vi "TETRIX Servos Move All_HT_myRIO.vi"(0 "Servo 4 (0 - 255)":u8(slide)=128 step=1 scale=0.0..255.0, 1 "Servo 5 (0 - 255)":u8(slide)=128 step=1 scale=0.0..255.0, 2 "Servo 6 (0 - 255)":u8(slide)=128 step=1 scale=0.0..255.0, 4 "Enable Sync: Fast | Medium | Slow | None":string(combo)="None", 5 "Controller Daisy Chain Position (1 - 4)":u8=1, 6 "Servo 3 (0 - 255)":u8(slide)=128 step=1 scale=0.0..255.0, 7 "Servo 2 (0 - 255)":u8(slide)=128 step=1 scale=0.0..255.0, 8 "Servo 1 (0 - 255)":u8(slide)=128 step=1 scale=0.0..255.0, 9 "error in (no error)":errorcluster) -> (3 "error out":errorcluster)   [LabVIEW 2014]
uses:
  <vilib>/myRIO/Instrument Drivers/Onboard IO/I2C/vis/Configure.vi
  <vilib>/myRIO/Instrument Drivers/Onboard IO/I2C/vis/Write.vi
  Global Servo Controls.vi
  <vilib>/myRIO/Instrument Drivers/Onboard IO/I2C/vis/Smart Open.vi
  <vilib>/Utility/error.llb/Error Cluster From Error Code.vi
  <vilib>/myRIO/Common/Instrument Driver Framework/myRIO v1.0/I2C/vis/myRIO v1.0 Configure I2C.vi
  <vilib>/myRIO/Common/Instrument Driver Framework/myRIO v1.0/I2C/vis/myRIO v1.0 Write I2C.vi
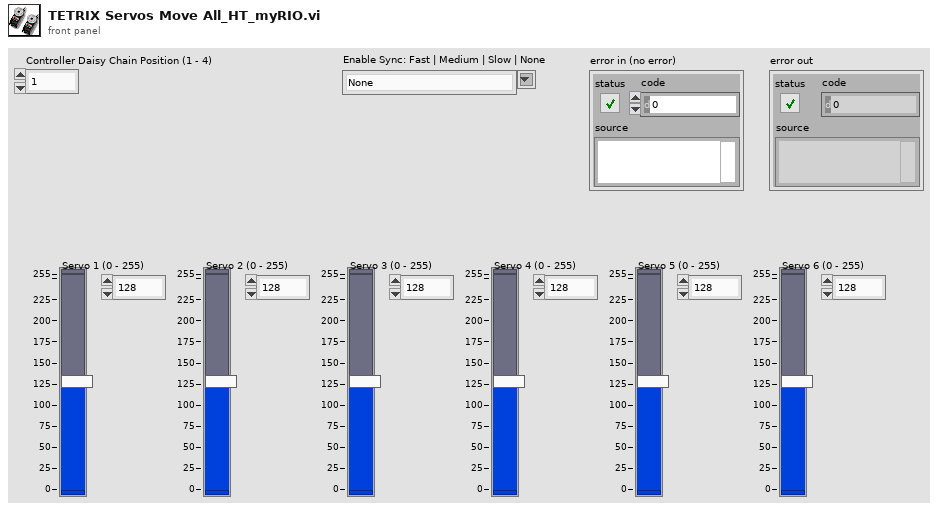
[diagram p1: front panel]
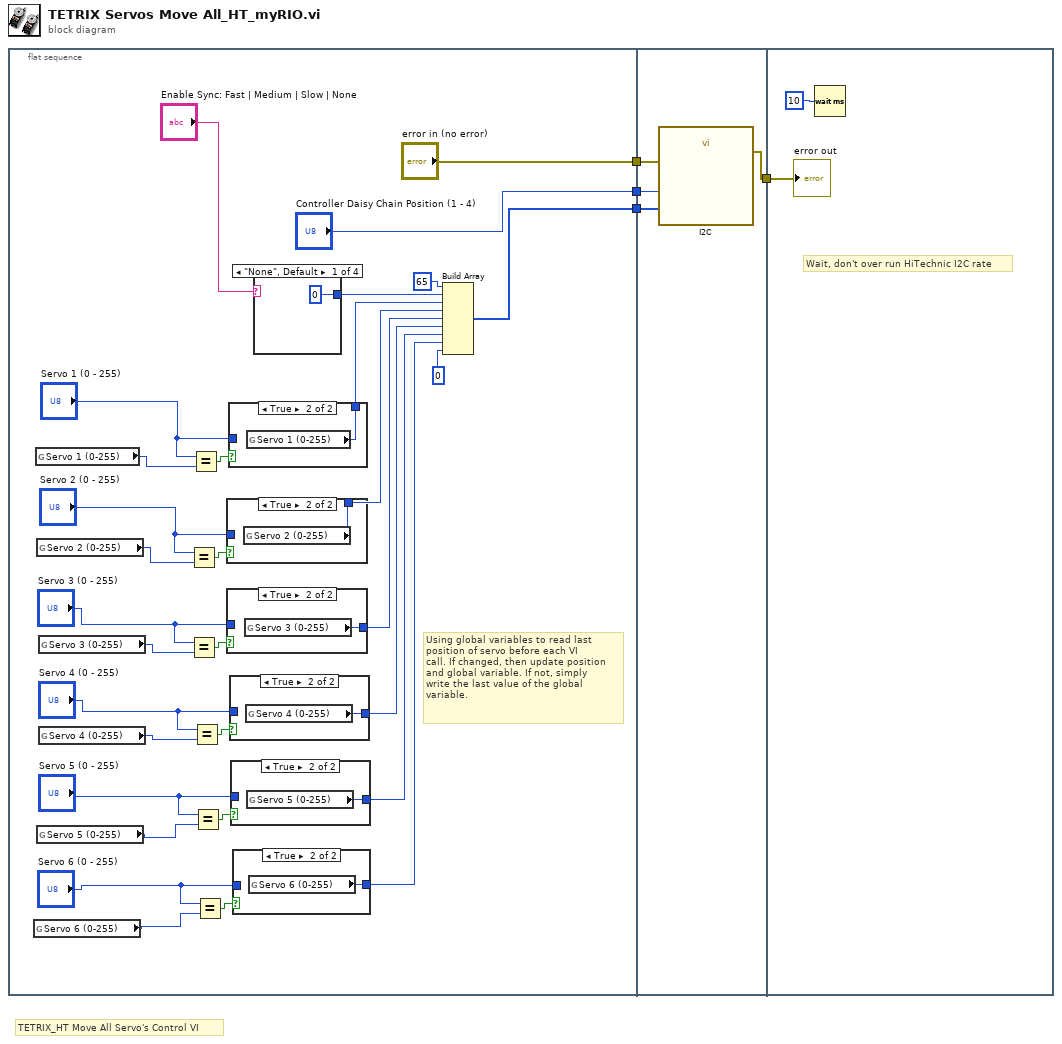
[diagram p0: block diagram]
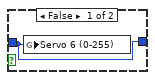
[diagram p2: hidden frame]
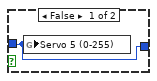
[diagram p3: hidden frame]
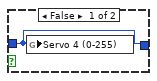
[diagram p4: hidden frame]
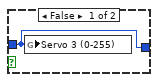
[diagram p5: hidden frame]
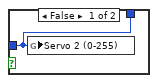
[diagram p6: hidden frame]
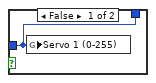
[diagram p7: hidden frame]
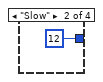
[diagram p8: hidden frame]
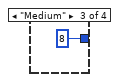
[diagram p9: hidden frame]
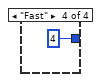
[diagram p10: hidden frame]
diagram:
  # "TETRIX_HT Move All Servo's Control VI"
  n1 = flat-sequence {
    tunnel: ["error in (no error)"] -> w4
    tunnel: ["Controller Daisy Chain Position (1 - 4)"] -> w3
    tunnel: [w29] -> w2
    tunnel: w4 -> [w55]
    tunnel: w3 -> [w54]
    tunnel: w2 -> [w53]
    tunnel: [w52] -> w1
    tunnel: w1 -> [w56]
    frame #0 {
      # "Using global variables to read last\nposition of servo before each VI\ncall. If changed, then update position\nand global variable. If not, simply\nwrite the last value of the global\nvariable."
      n2 = global read "Global Servo Controls.vi" "Servo 6 (0-255)"() -> (w14:u8)
      n3 = global read "Global Servo Controls.vi" "Servo 1 (0-255)"() -> (w10:u8)
      n4 = global read "Global Servo Controls.vi" "Servo 2 (0-255)"() -> (w18:u8)
      n5 = global read "Global Servo Controls.vi" "Servo 5 (0-255)"() -> (w15:u8)
      n6 = global read "Global Servo Controls.vi" "Servo 3 (0-255)"() -> (w17:u8)
      n7 = global read "Global Servo Controls.vi" "Servo 4 (0-255)"() -> (w16:u8)
      n8 = Equal?(x="Servo 2 (0 - 255)", y=w18) -> (x = y?=w27:bool)
      n9 = Equal?(x="Servo 3 (0 - 255)", y=w17) -> (x = y?=w26:bool)
      n10 = Equal?(x="Servo 1 (0 - 255)", y=w10) -> (x = y?=w28:bool)
      n11 = Equal?(x="Servo 4 (0 - 255)", y=w16) -> (x = y?=w24:bool)
      n12 = Equal?(x="Servo 5 (0 - 255)", y=w15) -> (x = y?=w22:bool)
      n13 = Equal?(x="Servo 6 (0 - 255)", y=w14) -> (x = y?=w20:bool)
      n14 = case shown="True" w27 {
        tunnel: "Servo 2 (0 - 255)" -> [w44 _]
        tunnel: [w44 w45] -> w9
        frame False {
          n15 = global write "Global Servo Controls.vi" "Servo 2 (0-255)"(w44) -> ()
        }
        frame True {
          n16 = global read "Global Servo Controls.vi" "Servo 2 (0-255)"() -> (w45:u8)
        }
      }
      n17 = case shown="True" w26 {
        tunnel: "Servo 3 (0 - 255)" -> [w42 _]
        tunnel: [w42 w43] -> w8
        frame False {
          n18 = global write "Global Servo Controls.vi" "Servo 3 (0-255)"(w42) -> ()
        }
        frame True {
          n19 = global read "Global Servo Controls.vi" "Servo 3 (0-255)"() -> (w43:u8)
        }
      }
      n20 = case shown="True" w28 {
        tunnel: "Servo 1 (0 - 255)" -> [w46 _]
        tunnel: [w46 w47] -> w11
        frame False {
          n21 = global write "Global Servo Controls.vi" "Servo 1 (0-255)"(w46) -> ()
        }
        frame True {
          n22 = global read "Global Servo Controls.vi" "Servo 1 (0-255)"() -> (w47:u8)
        }
      }
      n23 = case shown="True" w24 {
        tunnel: "Servo 4 (0 - 255)" -> [w40 _]
        tunnel: [w40 w41] -> w7
        frame False {
          n24 = global write "Global Servo Controls.vi" "Servo 4 (0-255)"(w40) -> ()
        }
        frame True {
          n25 = global read "Global Servo Controls.vi" "Servo 4 (0-255)"() -> (w41:u8)
        }
      }
      n26 = case shown="True" w22 {
        tunnel: "Servo 5 (0 - 255)" -> [w38 _]
        tunnel: [w38 w39] -> w6
        frame False {
          n27 = global write "Global Servo Controls.vi" "Servo 5 (0-255)"(w38) -> ()
        }
        frame True {
          n28 = global read "Global Servo Controls.vi" "Servo 5 (0-255)"() -> (w39:u8)
        }
      }
      n29 = case shown="True" w20 {
        tunnel: "Servo 6 (0 - 255)" -> [w36 _]
        tunnel: [w36 w37] -> w5
        frame False {
          n30 = global write "Global Servo Controls.vi" "Servo 6 (0-255)"(w36) -> ()
        }
        frame True {
          n31 = global read "Global Servo Controls.vi" "Servo 6 (0-255)"() -> (w37:u8)
        }
      }
      n32 = case shown="\"None\", Default" "Enable Sync: Fast | Medium | Slow | None" {
        tunnel: [u8 0 u8 12 u8 8 u8 4] -> w33
        frame "None", Default {
        }
        frame "Slow" {
        }
        frame "Medium" {
        }
        frame "Fast" {
        }
      }
      n33 = Build Array(u8 65 ("element"), w33, w11, w9, w8, w7, w6, w5, u8 0 ("element")) -> (w29:u8[])
    }
    frame #1 {
      n34 = call "I2C"("Slave Address (7-bit)"=w54, "Bytes to Write"=w53, "error in (no error)"=w55) -> ("error out"=w52:errorcluster)  [unwired: 24 in]
    }
    frame #2 {
      # "Wait, don't over run HiTechnic I2C rate"
      n35 = Wait (ms)(milliseconds to wait=u32 10) -> ()  [unwired: 1 out]
      "error out" <- w56
    }
  }
